vi "DIOLEDUpdate.vi"(2 "DIO LED Mode":T3, 3 "DIOLEDDevRefIn":T1={"DIO Channel"=enum."Invalid", "DevStatus"={"status"=FALSE, "code"=0, "source"=""}}) -> (1 "DIOLEDDevRefOut":T1={"DIO Channel"=enum."Invalid", "DevStatus"={"status"=FALSE, "code"=0, "source"=""}})   [LabVIEW 2018]
uses:
  TypeDefs/DIOLEDMode.ctl
  <vilib>/Rock Robotics/WPI/DigitalOutput/WPI_DigitalOutputDevRef.ctl
  <vilib>/Rock Robotics/SystemInterfaces/DIO/FPGA_DIOChannel.ctl
panel:
  in  "SlowBlinkPeriod (ms)":u16=2000
  in  "FastBlinkPeriod (ms)":u16=500
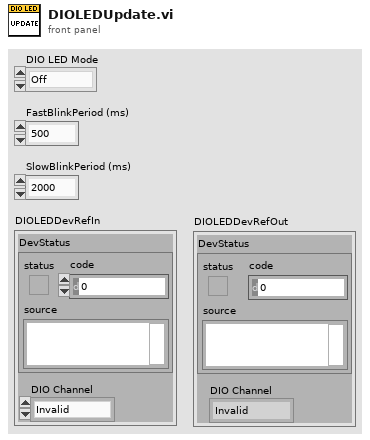
[diagram p1: front panel]
types:
  T1 = typedef "WPI_DigitalOutputDevRef.ctl" = cluster{"DIO Channel":T2, "DevStatus":errorcluster}
  T2 = typedef "FPGA_DIOChannel.ctl" = enum8{"DIO 0", "DIO 1", "DIO 2", "DIO 3", "DIO 4", "DIO 5", "DIO 6", "DIO 7", "DIO 8", "DIO 9", "DIO MXP 0", "DIO MXP 1", "DIO MXP 2", "DIO MXP 3", "DIO MXP 4", "DIO MXP 5", "DIO MXP 6", "DIO MXP 7", "DIO MXP 8", "DIO MXP 9", "DIO MXP 10", "DIO MXP 11", "DIO MXP 12", "DIO MXP 13", "DIO MXP 14", "DIO MXP 15", "SPI Port CS1", "SPI Port CS2", "SPI Port CS3", "SPI Port MISO", "SPI Port MOSI", "Invalid"}
  T3 = typedef "DIOLEDMode.ctl" = enum16{"Off", "On", "FastBlink", "SlowBlink"}
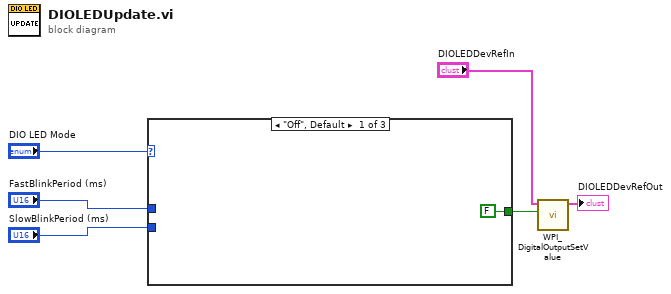
[diagram p0: block diagram]
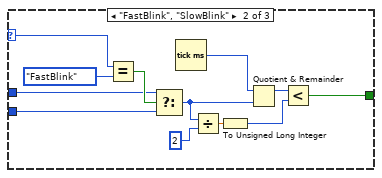
[diagram p2: hidden frame]
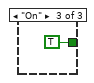
[diagram p3: hidden frame]
diagram:
  n1 = case shown="\"Off\", Default" "DIO LED Mode" {
    selector: "DIO LED Mode" -> [_ w19 _]
    tunnel: [FALSE ("Value") w8 TRUE ("Value")] -> w4
    tunnel: "FastBlinkPeriod (ms)" -> [_ w16 _]
    tunnel: "SlowBlinkPeriod (ms)" -> [_ w15 _]
    frame "Off", Default {
    }
    frame "FastBlink", "SlowBlink" {
      n2 = Equal?(x=w19, y=DIOLEDMode."FastBlink") -> (x = y?=w17:bool)
      n3 = Select(t=w16, s=w17, f=w15) -> (s? t:f=w10:u16)
      n4 = Tick Count (ms)() -> (millisecond timer value=w13:u32)
      n5 = Divide(x=w10, y=u16 2) -> (x/y=w12:sgl)
      n6 = To Unsigned Long Integer(number=w12) -> (unsigned 32bit integer=w9:u32)
      n7 = Quotient & Remainder(x=w13, y=w10) -> (x-y*floor(x/y)=w11:u32)  [unwired: 1 out]
      n8 = Less?(x=w11, y=w9) -> (x < y?=w8:bool)
    }
    frame "On" {
    }
  }
  n9 = call <vilib>:"WPI_DigitalOutputSetValue.vi"("Value"=w4, "DigitalOutputDevRef"="DIOLEDDevRefIn") -> ("DigitalOutputDevRef"=→"DIOLEDDevRefOut":T1)  [unwired: 8 in, 1 out]
